vi "write_attributes.vi"(8 "error in (no error)":errorcluster, 10 "attributes":T1, 11 "MultiTaskElasticNet in":refnum<class "MultiTaskElasticNet.lvclass">) -> (0 "error out":errorcluster, 3 "MultiTaskElasticNet out":refnum<class "MultiTaskElasticNet.lvclass">)   [LabVIEW 2020, in "MultiTaskElasticNet.lvclass"]
uses:
  MultiTaskElasticNet.lvclass
  Controls/multi_task_elastic_net_attributes.ctl
  MultiTaskElasticNet.lvclass/MultiTaskElasticNet.ctl
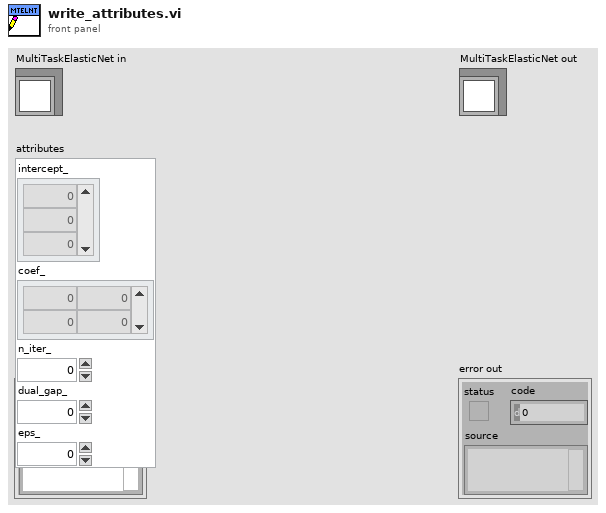
[diagram p1: front panel]
types:
  T1 = typedef "multi_task_elastic_net_attributes.ctl" = cluster{"intercept_":dbl[], "coef_":dbl[][], "n_iter_":dbl, "dual_gap_":dbl, "eps_":dbl}
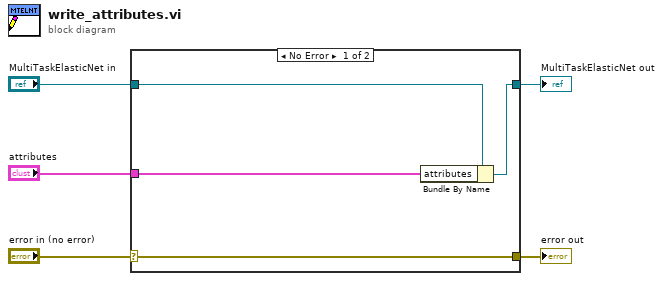
[diagram p0: block diagram]
diagram:
  n1 = case shown="No Error" "error in (no error)" {
    selector: "error in (no error)" -> [w9 w10]
    tunnel: [w9 w10] -> w4
    tunnel: [w7 w11] -> w2
    tunnel: "MultiTaskElasticNet in" -> [w8 w11]
    tunnel: "attributes" -> [w6 _]
    frame No Error {
      n2 = Bundle By Name(cluster=w8, "attributes"=w6) -> (w7:refnum<class "MultiTaskElasticNet.lvclass">)
    }
    frame Error {
    }
  }
  "error out" <- w4
  "MultiTaskElasticNet out" <- w2
